vi "FTW-Connector-SpawnNewActor-Deprecated.vi"(0 "FTW Actor Connector Type":refnum<class "FTW-ActorConnector.lvclass">, 5 "Configuration":string="{\n  \"Identity\": \"ActorName\",\n  \"DebugEnableInboxLogging\": false,\n  \"DebugEnableJobLogging\": false,\n  \"InboxAddress\": \"inproc://*\",\n  \"DebugShowPanel\": false\n}", 7 "Actor VI Filepath":path, 9 "Timeout":i32=1000 format="%dmsec", 11 "error in":errorcluster) -> (4 "FTW Actor Connector":refnum<class "FTW-ActorConnector.lvclass">, 6 "Initialized Response":string, 8 "Instance Inbox Address":string, 15 "error out":errorcluster)   [LabVIEW 2013, in "FTW-ActorConnector.lvclass"]
doc: "This is the spawn new actor that was used for a while. It lacks the minimum strict inputs required to launch an actor."
uses:
  FTW-ActorConnector.lvclass
panel:
  # "Inputs"
  # "Outputs"
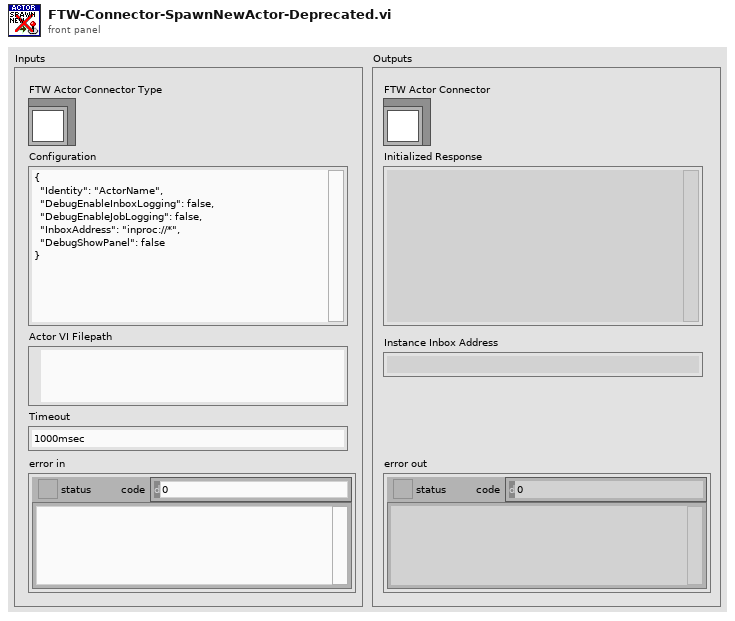
[diagram p1: front panel]
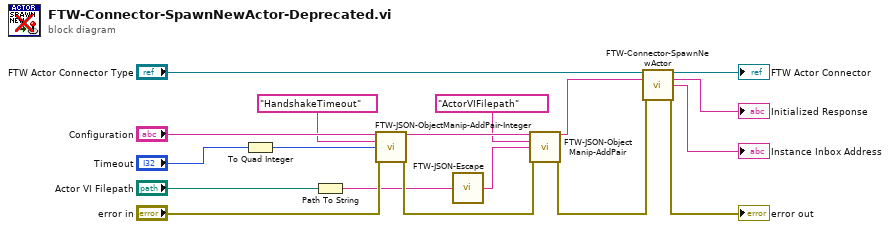
[diagram p0: block diagram]
diagram:
  n1 = To Quad Integer(1:"Timeout") -> (0:w9:i64)
  n2 = Path To String(path="Actor VI Filepath") -> (string=w2:string)
  n3 = call "FTW-JSON-ObjectManip-AddPair-Integer.vi"("Input JSON Object"="Configuration", "Key"="HandshakeTimeout", "Value"=w9, "error in"="error in") -> ("Output JSON Object"=w8:string, "error out"=w6:errorcluster)  [unwired: 10 in]
  n4 = call "FTW-JSON-Escape.vi"("String"=w2) -> ("Escaped UTF-8 String"=w1:string)
  n5 = call "FTW-JSON-ObjectManip-AddPair.vi"("Input JSON Object"=w8, "Key"="ActorVIFilepath", "Value"=w1, "error in"=w6) -> ("Output JSON Object"=w7:string, "error out"=w5:errorcluster)  [unwired: 10 in]
  n6 = call "FTW-Connector-SpawnNewActor.vi"("FTW Actor Connector Type"="FTW Actor Connector Type", "Configuration"=w7, "error in"=w5) -> ("FTW Actor Connector"=→"FTW Actor Connector":refnum<class "FTW-ActorConnector.lvclass">, "Initialized Response"=→"Initialized Response":string, "Instance Inbox Address"=→"Instance Inbox Address":string, "error out"=→"error out":errorcluster)  [unwired: 9 in]
